vi "Trigger Osc..vi"(9 "Source (0: Channel 1)":u16(ring) items=["Channel 1", "Channel 2", "Channel 3", "Channel 4", "Memory 1", "Memory 2", "Memory 3", "Memory 4", "Function 1", "Function 2", "Function 3", "Function 4", "Function 5", "Function 6", "Function 7", "Function 8"], 11 "VISA resource name":refnum<visa-resource-name>) -> (3 "Waveform Data":waveform(dbl)(graph))   [LabVIEW 2020]
doc: "This triggers the oscilloscope to fetch the current waveform being displayed on the oscilloscope on the specified channel. The model of the oscilloscope as well as the channel can be specified.\n\nArgs:\nVISA resource name - Specifies the model of the oscilloscope to be used (see user manual to add new model)\nSource - Channel to be read, (0 -> Channel 1, 1 -> Channel 2, etc.)\n\nReturns \nWaveform Data - The output data obtained from the trigger, i.e. the A-scan for that point"
uses:
  <instrlib>/LeCroy Wave Series/LeCroy Wave Series.lvlib
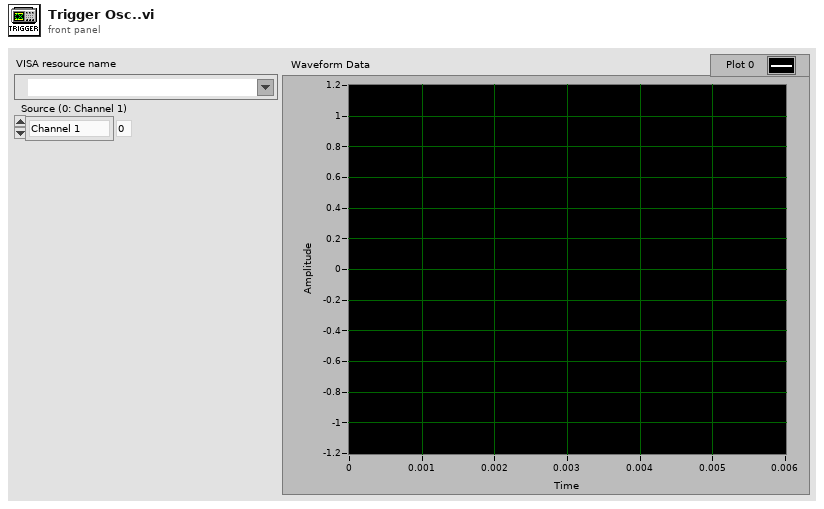
[diagram p1: front panel]
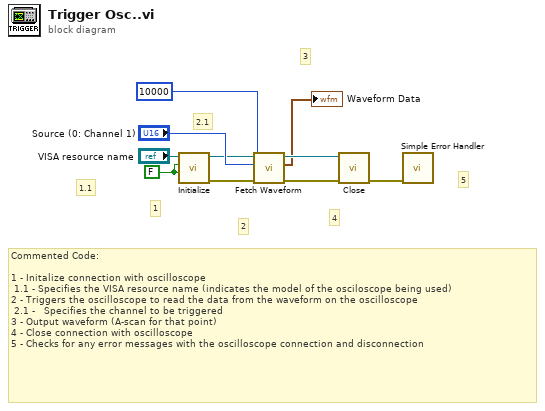
[diagram p0: block diagram]
diagram:
  w2 = FALSE ("Reset? (T: Yes)")
  # "5"
  # "3"
  # "4"
  # "2.1"
  # "2"
  # "1.1"
  # "1"
  # "Commented Code:\n\n1 - Initalize connection with oscilloscope\n 1.1 - Specifies the VISA resource name (indicates the model of the osciloscope being used)\n2 - Triggers the oscilloscope to read the data from the waveform on the oscilloscope \n 2.1 -   Specifies the channel to be triggered\n3 - Output waveform (A-scan for that point)\n4 - Close connection with oscilloscope\n5 - Checks for any error messages with the oscilloscope connection and disconnection"
  n1 = call <instrlib>:"Initialize.vi"("Reset? (T: Yes)"=w2, "ID Query? (T: Yes)"=w2, "VISA resource name"="VISA resource name") -> ("error out"=w4:errorcluster, "VISA resource name out"=w3:refnum<visa-resource-name>)  [unwired: 7 in]
  n2 = call <instrlib>:"Fetch Waveform.vi"("error in (no error)"=w4, "Timeout (10000 ms)"=u32 10000, "Source (0: Channel 1)"="Source (0: Channel 1)", "VISA resource name"=w3) -> ("error out"=w8:errorcluster, "Waveform Graph"=→"Waveform Data":waveform(dbl), "VISA resource name out"=w9:refnum<visa-resource-name>)  [unwired: 5 in]
  n3 = call <instrlib>:"Close.vi"("error in (no error)"=w8, "VISA resource name"=w9) -> ("error out"=w10:errorcluster)  [unwired: 9 in]
  n4 = call <vilib>:"Simple Error Handler.vi"("error in (no error)"=w10) -> ()  [unwired: 4 in, 5 out]
